vi "Abort Fit Global.vi"() -> ()   [LabVIEW 2021, in "Fits.lvlib"]
uses:
  Fits.lvlib
panel:
  out "Abort Fit":bool
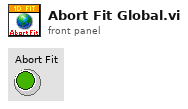
[diagram p1: front panel]
diagram:
